vi "Msg Send Response.vi"(5 "Response Notifier":refnum<notifier>, 6 "error in (no error)":errorcluster, 9 "response":variant) -> (0 "error out":errorcluster)   [LabVIEW 2014]
doc: "Sends a response to the original sender of a message (sent via Msg Send Message). It should form bookends with Msg Get Message in the message handling loop.\n\nThis is part of the Msg suite, intended to make messaging architectures in LabVIEW\nSee the template \"Message Based Application Template.vi\" for normal usage.\n\nCopyright 2005-2016 Jason Sommerville\n\nThis VI may be freely used, modified or distributed under the BSD license."
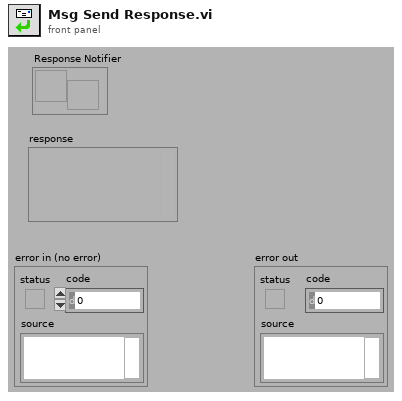
[diagram p1: front panel]
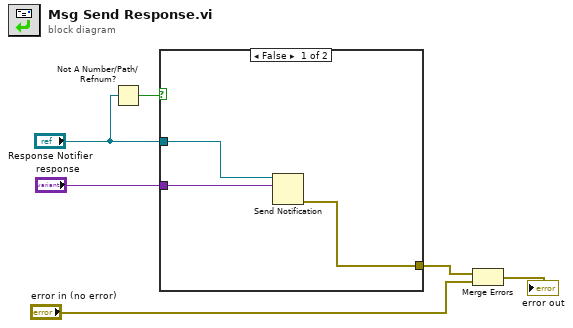
[diagram p0: block diagram]
diagram:
  n1 = Not A Number/Path/Refnum?(number/path/refnum="Response Notifier") -> (NaN/Path/Refnum?=w6:bool)
  n2 = case shown="False" w6 {
    tunnel: [w9 _] -> w4
    tunnel: "Response Notifier" -> [w8 _]
    tunnel: "response" -> [w7 _]
    frame False {
      n3 = Send Notification(notification=w7, notifier=w8) -> (error out=w9:errorcluster)  [unwired: 1 in, 1 out]
    }
    frame True {
    }
  }
  n4 = Merge Errors(w4, "error in (no error)") -> (→"error out":errorcluster)
